vi "(SubVI) Slowly Go to Target Posiiton_YCC-v2.vi"(4 "scan rate  (um/s)":dbl=2.0 format="%.3f", 5 "axis":u32=1, 6 "Target position (um)":dbl, 7 "Now position (um)":dbl) -> (1 "step size (nm)":dbl, 3 "True rate?":bool)   [LabVIEW 2014]
panel:
  out "traveling time (s)":dbl
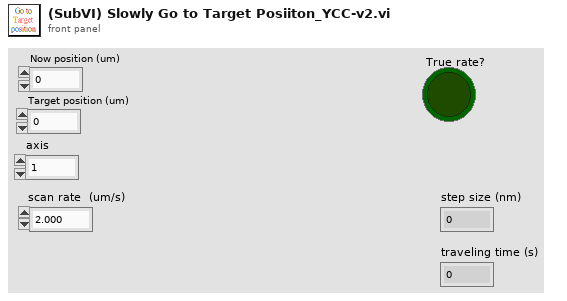
[diagram p1: front panel]
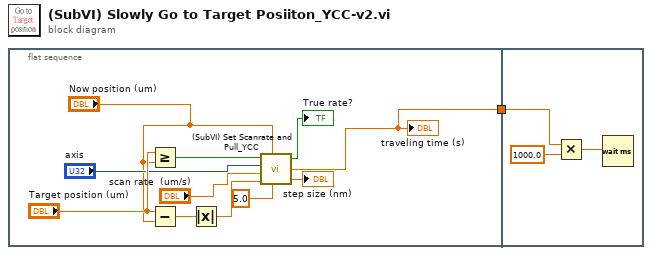
[diagram p0: block diagram]
diagram:
  n1 = flat-sequence {
    tunnel: [w3] -> w1
    tunnel: w1 -> [w13]
    frame #0 {
      n2 = Greater Or Equal?(x="Target position (um)", y="Now position (um)") -> (x >= y?=w12:bool)
      n3 = Subtract(x="Target position (um)", y="Now position (um)") -> (x-y=w10:dbl)
      n4 = Absolute Value(x=w10) -> (abs(x)=w9:dbl)
      n5 = call "(SubVI) Set Scanrate and Pull_YCC.vi"("toward+ ?\nT=+, F=-"=w12, "Start From  (um)"="Now position (um)", "axis"="axis", "scan rate  (um/s)"="scan rate  (um/s)", "waiting time per point (ms)\nrange from 5ms to 0.167 ms"=5.0 ("waiting time per point (ms)\nrange from 5ms to 0.167 ms"), "range  (um)"=w9) -> ("True rate?"=→"True rate?":bool, "traveling time (s)"=w3:dbl, "step size (nm)"=→"step size (nm)":dbl)
      "traveling time (s)" <- w3
    }
    frame #1 {
      n6 = Multiply(x=w13, y=1000.0) -> (x*y=w15:dbl)
      n7 = Wait (ms)(milliseconds to wait=w15) -> ()  [unwired: 1 out]
    }
  }
